vi "AutoRecycleBinToFeeder.vi"(8 "error in (no error)":errorcluster) -> ()   [LabVIEW 2014]
uses:
  <vilib>/Rock Robotics/WPI/DriverStation/WPI_DriverStationRobotMode2.ctl
  Robot Global Data.vi
  AutomationGlobals.vi
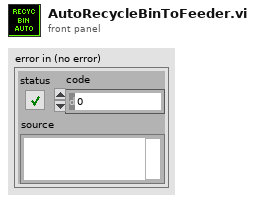
[diagram p1: front panel]
types:
  T1 = typedef "WPI_DriverStationRobotMode2.ctl" = enum16{"Autonomous Disabled", "Autonomous Enabled", "Teleop Disabled", "Teleop Enabled", "Disconnected", "Finish", "Test Disabled", "Test Enabled", "Emergency Stopped"}
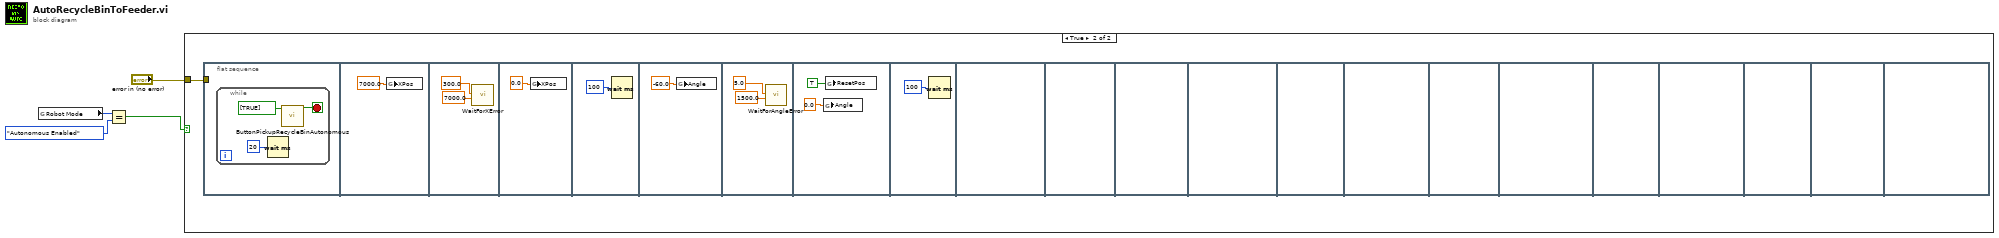
[diagram p0: block diagram]
diagram:
  n1 = global read "Robot Global Data.vi" "Robot Mode"() -> (w3:T1)
  n2 = Equal?(x=w3, y=WPI_DriverStationRobotMode2."Autonomous Enabled") -> (x = y?=w1:bool)
  n3 = case shown="True" w1 {
    tunnel: "error in (no error)" -> [_ w5]
    frame False {
    }
    frame True {
      n4 = flat-sequence {
        tunnel: w5 -> [_]
        frame #0 {
          n5 = while {
            stop <- w6 stop-if-true
            n6 = Wait (ms)(milliseconds to wait=u32 20) -> ()  [unwired: 1 out]
            n7 = call "ButtonPickupRecycleBinAutonomous.vi"("Buttons"=bool[] [TRUE]) -> ("Boolean"=w6:bool)  [unwired: 10 in]
          }
        }
        frame #1 {
          n8 = global write "AutomationGlobals.vi" "XPos"(7000.0 ("XPos")) -> ()
        }
        frame #2 {
          n9 = call "WaitForXError.vi"("Timeout (ms)"=7000.0, "AllowedError"=300.0) -> ()  [unwired: 9 in, 1 out]
        }
        frame #3 {
          n10 = global write "AutomationGlobals.vi" "XPos"(0.0 ("XPos")) -> ()
        }
        frame #4 {
          n11 = Wait (ms)(milliseconds to wait=u32 100) -> ()  [unwired: 1 out]
        }
        frame #5 {
          n12 = global write "AutomationGlobals.vi" "Angle"(-60.0 ("XPos")) -> ()
        }
        frame #6 {
          n13 = call "WaitForAngleError.vi"("Timeout (ms)"=1500.0, "AllowedError"=5.0) -> ()  [unwired: 9 in, 1 out]
        }
        frame #7 {
          n14 = global write "AutomationGlobals.vi" "Angle"(0.0 ("XPos")) -> ()
          n15 = global write "AutomationGlobals.vi" "ResetPos"(TRUE ("ResetGyro")) -> ()
        }
        frame #8 {
          n16 = Wait (ms)(milliseconds to wait=u32 100) -> ()  [unwired: 1 out]
        }
        frame #9 {
        }
        frame #10 {
        }
        frame #11 {
        }
        frame #12 {
        }
        frame #13 {
        }
        frame #14 {
        }
        frame #15 {
        }
        frame #16 {
        }
        frame #17 {
        }
        frame #18 {
        }
        frame #19 {
        }
        frame #20 {
        }
        frame #21 {
        }
      }
    }
  }
